vi "Acquire-c.vi"() -> (0 "Waveform Chart":dbl[](graph))   [LabVIEW 2020]
uses:
  Typedefs/Stop cases.ctl
panel:
  out "Error out":errorcluster
  in  "Error in":errorcluster
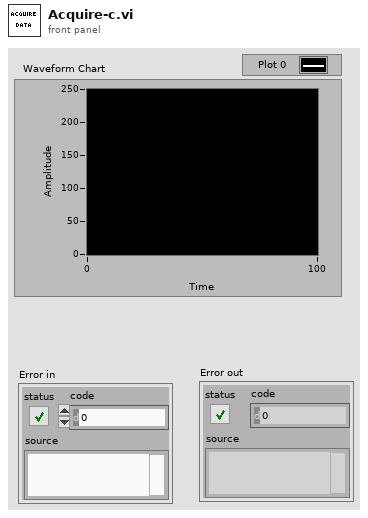
[diagram p1: front panel]
types:
  T1 = typedef "Stop cases.ctl" = enum16{"Initialize", "Write", "Stop"}
  T2 = enum16{"Initialize", "Enqueue", "Dequeue", "Sum"}
  T3 = enum32{"Bad", "Idle", "Run top level", "Running"}
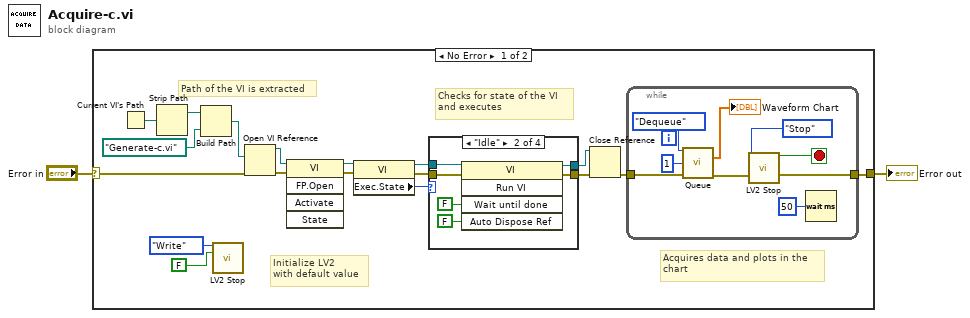
[diagram p0: block diagram]
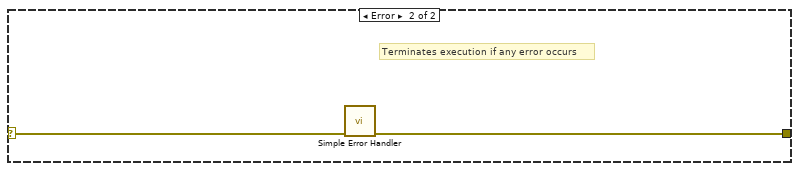
[diagram p5: hidden frame]
diagram:
  n1 = case shown="No Error" "Error in" {
    selector: "Error in" -> [w12 w43]
    tunnel: [w5 w42] -> w1
    frame No Error {
      # "Acquires data and plots in the \nchart"
      # "Checks for state of the VI \nand executes"
      # "Path of the VI is extracted"
      # "Initialize LV2 \nwith default value"
      n2 = Current VI's Path() -> (path=w20:path)
      n3 = Strip Path(path=w20) -> (stripped path=w19:path)  [unwired: 1 out]
      n4 = Build Path(base path=w19, name or relative path=path "Generate-c.vi") -> (appended path=w17:path)
      n5 = call "LV2 Stop.vi"("Operation"=Stop_cases."Write", "Stop"=FALSE) -> ()  [unwired: 12 in, 2 out]
      n6 = Open VI Reference(vi path=w17, error in (no error)=w12) -> (vi reference=w15:refnum<vi>, error out=w16:errorcluster)  [unwired: 4 in]
      n7 = invoke class="VI" method="FP.Open"(reference=w15, error in=w16) -> (reference out=w14:refnum<vi>, error out=w13:errorcluster)  [unwired: 3 in, 3 out]
      n8 = property class="VI"(reference=w14, error in=w13) -> (reference out=w10:refnum<vi>, error out=w9:errorcluster, "Exec.State"=w11:T3)
      n9 = case shown="\"Idle\"" w11 {
        tunnel: w10 -> [w22 w28 w30 w32]
        tunnel: w9 -> [w21 w27 w29 w31]
        tunnel: [w21 w24 w29 w31] -> w8
        tunnel: [w22 w23 w30 w32] -> w7
        frame "Bad" {
        }
        frame "Idle" {
          n10 = invoke class="VI" method="Run VI"(reference=w28, error in=w27, "Wait until done"=FALSE ("Wait Until Done"), "Auto Dispose Ref"=FALSE ("Auto Dispose Reference")) -> (reference out=w23:refnum<vi>, error out=w24:errorcluster)  [unwired: 1 in, 3 out]
        }
        frame "Run top level" {
        }
        frame "Running" {
        }
      }
      n11 = Close Reference(reference=w7, error in (no error)=w8) -> (error out=w6:errorcluster)
      n12 = while {
        tunnel: w6 -> [w41]
        tunnel: [w39] -> w5
        stop <- w36 stop-if-true
        n13 = call "Queue.vi"("Operation"=T2."Dequeue", "Size"=1, "Error in"=w41) -> ("Dequeue"=→"Waveform Chart":dbl[], "Error out"=w40:errorcluster)  [unwired: 7 in, 4 out]
        n14 = call "LV2 Stop.vi"("Operation"=Stop_cases."Stop", "Error in"=w40) -> ("Output"=w36:bool, "Error out"=w39:errorcluster)  [unwired: 12 in]
        n15 = Wait (ms)(milliseconds to wait=u32 50) -> ()  [unwired: 1 out]
      }
    }
    frame Error {
      # "Terminates execution if any error occurs"
      n16 = call <vilib>:"Simple Error Handler.vi"("error in (no error)"=w43) -> ("error out"=w42:errorcluster)  [unwired: 4 in, 4 out]
    }
  }
  "Error out" <- w1
